vi "Read Measurement Method.vi"(6 "wait for reply (T)":bool=TRUE, 8 "error in":errorcluster, 9 "Measurement Type (0: Frequency)":i32(ring) items=["Frequency", "Mean", "Period", "Pulse Duty", "Peak to Peak", "Cycle RMS", "Minimum", "Maximum", "Rise Time", "Fall Time", "Positive Width", "Negative Width", "Amplitude", "Cycle Mean", "High", "Low", "Negative Duty", "Positive Overshoot", "Negative Overshoot", "Cursor Mean", "Burst Width", "Positive Pulse Count", "Negative Pulse Count", "Rising Edge Count", "Falling Edge Count", "Area", "Cycle Area", "RMS", "Cursor RMS"], 10 "Channel (1: Channel 1)":i32(ring)=1 items=["Channel 1"=1, "Channel 2"=2, "Channel 3"=3, "Channel 4"=4], 11 "Module ID":i32=-1) -> (0 "error out":errorcluster, 1 "timed out?":bool, 2 "Measurement":dbl, 3 "Units":string)   [LabVIEW 2020, in "Osciloscope.lvlib"]
doc: "_____\nCreated using DQMH Event Scripter 6.0.0.122."
uses:
  Osciloscope.lvlib
  Read Measurement Method Argument--cluster.ctl
  Read Measurement Method (Reply Payload)--cluster.ctl
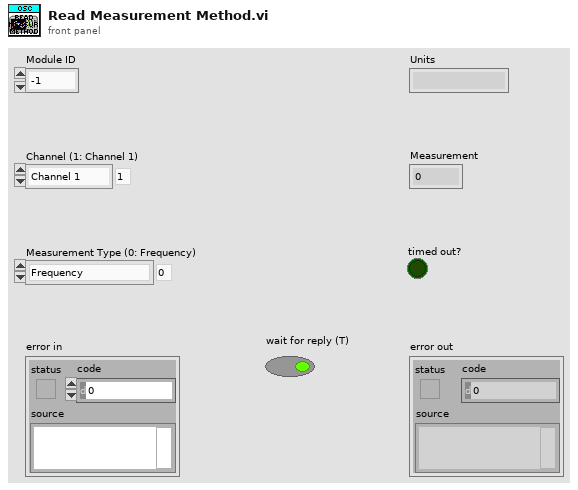
[diagram p1: front panel]
types:
  T1 = typedef "Osciloscope.lvlib/Read Measurement Method Argument--cluster.ctl" = cluster{"Module ID":i32, "Channel (1: Channel 1)":i32, "Measurement Type (0: Frequency)":i32, "Wait Notifier":refnum<notifier>, "wait for reply":bool}
  T2 = typedef "Osciloscope.lvlib/Request Events--cluster.ctl" = cluster{"Stop Module":refnum<user-event>, "Show Panel":refnum<user-event>, "Hide Panel":refnum<user-event>, "Show Diagram":refnum<user-event>, "Get Module Execution Status":refnum<user-event>, "Set Port Com":refnum<user-event>, "InicializarOsciloscopio":refnum<user-event>, "InitMethod":refnum<user-event>, "CloseMethod":refnum<user-event>, "MethodAutosetup":refnum<user-event>, "Method Configure Channel":refnum<user-event>, "Reset Method":refnum<user-event>, "Read WAVEFORM Method":refnum<user-event>, "Read measurement method":refnum<user-event>, "Read 2 channels measurement":refnum<user-event>}
  T3 = typedef "Osciloscope.lvlib/Read Measurement Method (Reply Payload)--cluster.ctl" = cluster{"Units":string, "Measurement":dbl, "Read measurement method_error":errorcluster}
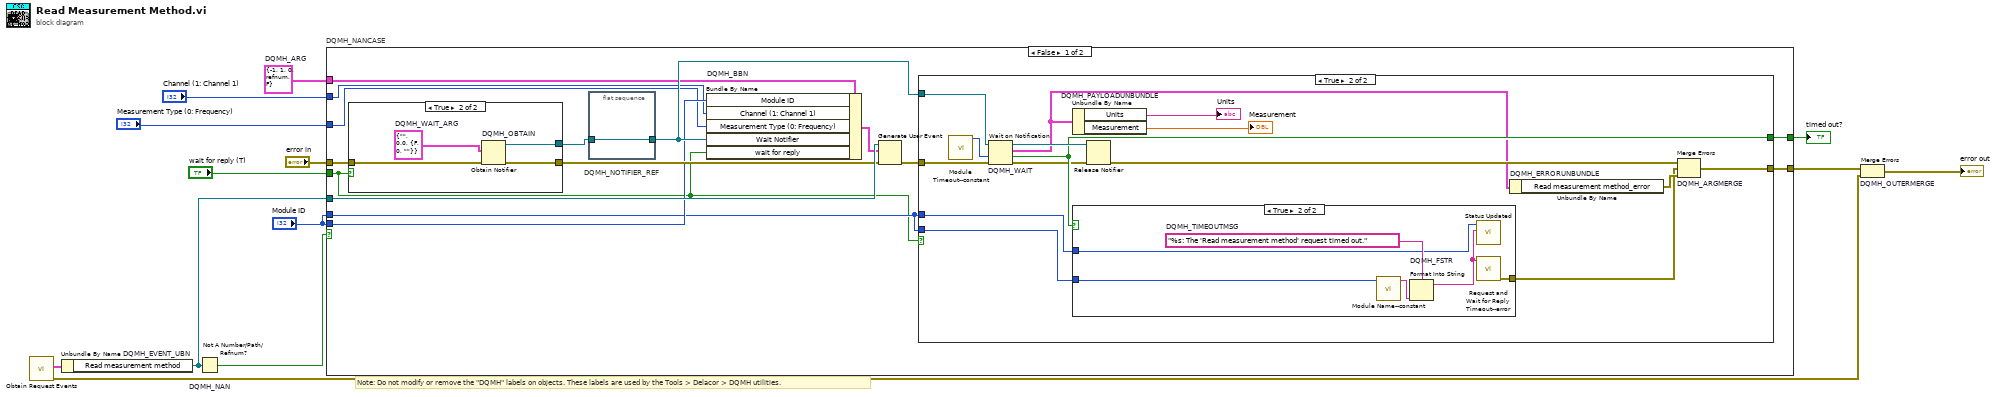
[diagram p0: block diagram]
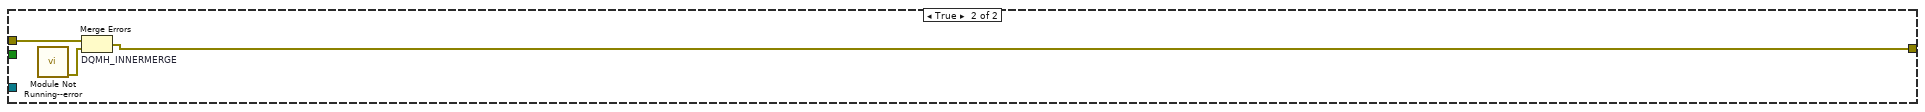
[diagram p5: hidden frame]
diagram:
  w7 = T1 {"Module ID"=-1, "Channel (1: Channel 1)"=1, "Measurement Type (0: Frequency)"=0, "Wait Notifier"=refnum, "wait for reply"=FALSE}  # DQMH_ARG
  # "Note: Do not modify or remove the \"DQMH\" labels on objects. These labels are used by the Tools > Delacor > DQMH utilities."
  n1 = call "Obtain Request Events.vi"() -> ("error out"=w2:errorcluster, "Osciloscope Request Events"=w1:T2)  [unwired: 10 in]
  n2 = Unbundle By Name "DQMH_EVENT_UBN"(w1) -> ("Read measurement method"=w11:refnum<user-event>)
  n3 = Not A Number/Path/Refnum? "DQMH_NAN"(number/path/refnum=w11) -> (NaN/Path/Refnum?=w10:bool)
  n4 = case "DQMH_NANCASE" shown="False" w10 {
    tunnel: "error in" -> [w28 w59]
    tunnel: w11 -> [w26 _]
    tunnel: [w23 w58] -> w8
    tunnel: [w24 _] -> w9
    tunnel: w7 -> [w19 _]
    tunnel: "Module ID" -> [w18 _]
    tunnel: "Channel (1: Channel 1)" -> [w17 _]
    tunnel: "Measurement Type (0: Frequency)" -> [w16 _]
    tunnel: "Module ID" -> [w15 _]
    tunnel: "wait for reply (T)" -> [w14 _]
    frame False {
      n5 = case shown="True" w14 {
        tunnel: w28 -> [w52 w56]
        tunnel: [w52 w55] -> w25
        tunnel: [_ w53] -> w21
        frame False {
        }
        frame True {
          w54 = T3 {"Units"="", "Measurement"=0.0, "Read measurement method_error"={"status"=FALSE, "code"=0, "source"=""}}  # DQMH_WAIT_ARG
          n6 = Obtain Notifier "DQMH_OBTAIN"(notification data type=w54, error in (no error)=w56) -> (notifier out=w53:refnum<notifier>, error out=w55:errorcluster)  [unwired: 2 in, 1 out]
        }
      }
      n7 = flat-sequence "DQMH_NOTIFIER_REF" {
        tunnel: w21 -> [w29]
        tunnel: [w29] -> w20
        frame #0 {
        }
      }
      n8 = Bundle By Name "DQMH_BBN"(cluster=w19, "Module ID"=w18, "Channel (1: Channel 1)"=w17, "Measurement Type (0: Frequency)"=w16, "Wait Notifier"=w20, "wait for reply"=w14) -> (w22:T1)
      n9 = Generate User Event(user event=w26, event data cluster=w22, error in=w25) -> (error out=w27:errorcluster)  [unwired: 1 in, 1 out]
      n10 = case shown="True" w14 {
        tunnel: w27 -> [w30 w45]
        tunnel: w20 -> [_ w44]
        tunnel: [_ w42] -> w24
        tunnel: [w30 w41] -> w23
        tunnel: w15 -> [_ w32]
        tunnel: w15 -> [_ w31]
        frame False {
        }
        frame True {
          n11 = call "Module Timeout--constant.vi"() -> ("Module Timeout"=w35:i32)  [unwired: 11 in]
          n12 = Wait on Notification "DQMH_WAIT"(notifier=w44, timeout in ms (-1)=w35, error in (no error)=w45) -> (notifier out=w43:refnum<notifier>, notification=w36:T3, timed out?=w42:bool, error out=w40:errorcluster)  [unwired: 1 in]
          n13 = Unbundle By Name "DQMH_PAYLOADUNBUNDLE"(w36) -> ("Units"=→"Units":string, "Measurement"=→"Measurement":dbl)
          n14 = case shown="True" w42 {
            tunnel: [_ w49] -> w37
            tunnel: w32 -> [_ w47]
            tunnel: w31 -> [_ w46]
            frame False {
            }
            frame True {
              w51 = "%s: The 'Read measurement method' request timed out."  # DQMH_TIMEOUTMSG
              n15 = call "Module Name--constant.vi"("Module ID"=w46) -> ("Module Name"=w48:string)  [unwired: 10 in]
              n16 = Format Into String "DQMH_FSTR"(format string=w51, w48) -> (resulting string=w50:string)  [unwired: 2 in, 1 out]
              n17 = call "Status Updated.vi"("Status"=w50, "Module ID"=w47) -> ()  [unwired: 9 in, 1 out]
              n18 = call "Request and Wait for Reply Timeout--error.vi"("Error Message"=w50) -> ("error out"=w49:errorcluster)  [unwired: 10 in]
            }
          }
          n19 = Release Notifier(notifier=w43, error in (no error)=w40) -> (error out=w39:errorcluster)  [unwired: 1 in, 2 out]
          n20 = Unbundle By Name "DQMH_ERRORUNBUNDLE"(w36) -> ("Read measurement method_error"=w38:errorcluster)
          n21 = Merge Errors "DQMH_ARGMERGE"(w39, w37, w38) -> (w41:errorcluster)
        }
      }
    }
    frame True {
      n22 = call "Module Not Running--error.vi"() -> ("error out"=w57:errorcluster)  [unwired: 11 in]
      n23 = Merge Errors "DQMH_INNERMERGE"(w59, w57) -> (w58:errorcluster)
    }
  }
  "timed out?" <- w9
  n24 = Merge Errors "DQMH_OUTERMERGE"(w8, w2) -> (→"error out":errorcluster)
